vi "Write Meta Data (Serial Ref).vi"(6 "options":T1={"ignore timeout error"=TRUE, "timeout ms (1000)"=1000}, 7 "meta data":T2[](array[typedef]), 8 "error in":errorcluster, 11 "VISA resource name":refnum<visa-resource-name>) -> (0 "error out":errorcluster, 3 "connection info out":T3)   [LabVIEW 2010, in "NI STM.lvlib"]
doc: "Use this VI to transmit the meta data cluster to a remote computer. Sending the meta data to another computer helps maintainability since the data resides only on one side and it is shared to other computers at run time.\n\nCopyright 2015, 2016, 2017 National Instruments Corporation\n\nLicensed under the Apache License, Version 2.0 (the \"License\"); you may not use this file except in compliance with the License.\n\n You may obtain a copy of the License at\n\n http://www.apache.org/licenses/LICENSE-2.0\n\nUnless required by applicable law or agreed to in writing, software distributed under the License is distributed on an \"AS IS\" BASIS, WITHOUT WARRANTIES OR CONDITIONS OF ANY KIND, either express or implied.\n\nSee the License for the specific language governing permissions and limitations under the License."
uses:
  NI STM.lvlib
  Serial Connection Info.ctl
  SubVIs/MetaDataElement.ctl
  Serial Write Options.ctl
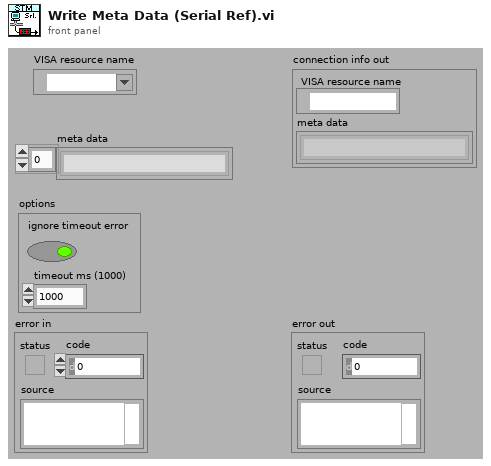
[diagram p1: front panel]
types:
  T1 = typedef "NI STM.lvlib/Serial Write Options.ctl" = cluster{"ignore timeout error":bool, "timeout ms (1000)":u32}
  T2 = typedef "NI STM.lvlib/MetaDataElement.ctl" = string
  T3 = typedef "NI STM.lvlib/Serial Connection Info.ctl" = cluster{"VISA resource name":refnum<visa-resource-name>, "meta data":T2[]}
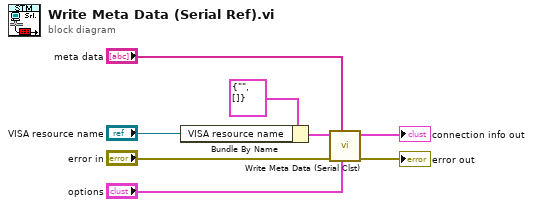
[diagram p0: block diagram]
diagram:
  n1 = Bundle By Name(cluster=T3 {"VISA resource name"="", "meta data"=[]} ("Connection Info Out"), "VISA resource name"="VISA resource name") -> (w1:T3)
  n2 = call "Write Meta Data (Serial Clst).vi"("options"="options", "meta data"="meta data", "error in"="error in", "connection info in"=w1) -> ("error out"=→"error out":errorcluster, "connection info out"=→"connection info out":T3)  [unwired: 6 in]
